vi "LEBITplc.DelayedDC.vi"(1 "i attribute":T1, 2 "Nickname":string="NDC6", 4 "Delayed DC":string[][](array[string]), 5 "Value":dbl, 8 "Enum":enum16{"RFAMP3", "Alpha", "DC"}(ring)) -> (14 "NicknamePDC":string, 15 "NicknameNDC":string, 16 "ValuePDC":dbl, 17 "IndexPDC":i32, 18 "ValueNDC":dbl, 19 "IndexNDC":i32)   [LabVIEW 2014, in "LEBITplc.lvlib"]
uses:
  LEBITplc.lvlib
  LEBITplc.i attribute.ctl
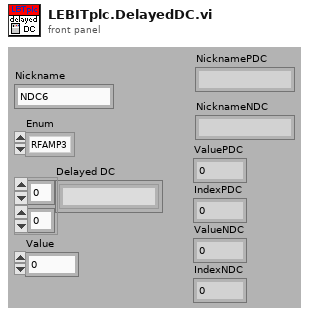
[diagram p1: front panel]
types:
  T1 = typedef "LEBITplc.lvlib/LEBITplc.i attribute.ctl" = cluster{"LLFLocation":string, "SetFileLocation":string, "nickNames":string[], "setValuePLCServiceID":i32[], "GUIServiceID":i32[], "monValuePLC":string[], "SetValueServiceID":i32[], "MonValueServiceID":i32[], "SetValue":dbl[][], "SetValueMin":dbl[], "SetValueMax":dbl[], "SetValueInfoServiceID":i32[], "GUINames":string[], "ListOfBases":string[], "Scale":dbl[], "Offset":dbl[], "setValuePLC":string[], "BaseName":string[], "ScaleServiceID":i32[], "OffsetServiceID":i32[], "AllPLCValues":string[], "CondSpecialArray":string[][], "CondSpecialIndex":i32[], "CondSpecialMonValue":dbl[], "RecentlyChanged":i32[], "SetFileLocationID":i32, "Dependent-Monitors":string[][], "LastLoadedFiles":string[], "IonGuideCalibLocation":string, "Monitor Dependent":string[], "Special":string[], "PLC?":bool[], "Start Date":string, "ListOfBasesServiceID":i32, "SETRA VISA resource":refnum<visa-resource-name>}
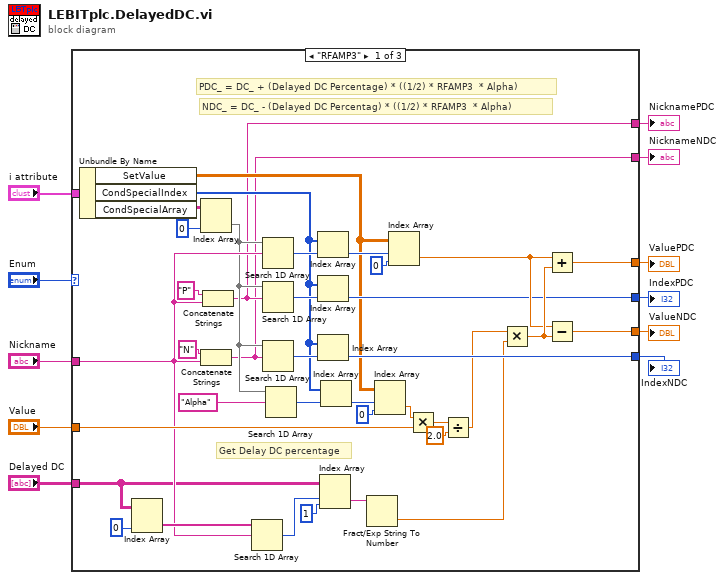
[diagram p0: block diagram]
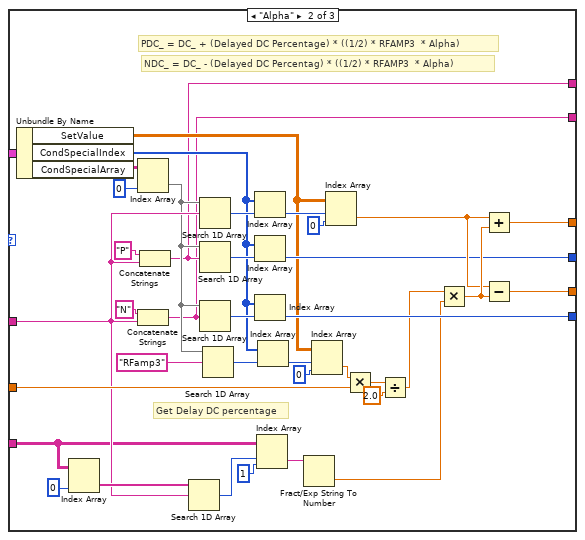
[diagram p2: hidden frame]
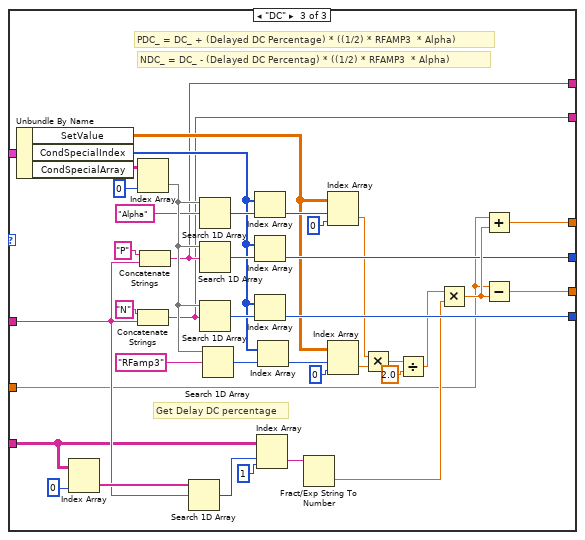
[diagram p3: hidden frame]
diagram:
  n1 = case shown="\"RFAMP3\"" "Enum" {
    tunnel: "Value" -> [w36 w74 w90]
    tunnel: [w40 w78 w118] -> w6
    tunnel: [w39 w77 w117] -> w7
    tunnel: [w38 w76 w116] -> w8
    tunnel: [w37 w75 w115] -> w9
    tunnel: "Nickname" -> [w28 w66 w107]
    tunnel: "i attribute" -> [w32 w70 w111]
    tunnel: "Delayed DC" -> [w27 w65 w106]
    tunnel: [w13 w51 w89] -> w2
    tunnel: [w12 w50 w88] -> w1
    frame "RFAMP3" {
      # "Get Delay DC percentage"
      # "NDC_ = DC_ - (Delayed DC Percentag) * ((1/2) * RFAMP3  * Alpha)"
      # "PDC_ = DC_ + (Delayed DC Percentage) * ((1/2) * RFAMP3  * Alpha)"
      n2 = Unbundle By Name(w32) -> ("SetValue"=w19:dbl[][], "CondSpecialIndex"=w23:i32[], "CondSpecialArray"=w31:string[][])
      n3 = Index Array(array=w27, index (col)=0 ("disabled index (col)")) -> (element=w29:string[])  [unwired: 1 in]
      n4 = Index Array(array=w31, index (col)=0 ("index (row)")) -> (element=w22:string[])  [unwired: 1 in]
      n5 = Concatenate Strings("N" ("string"), w28) -> (w12:string)
      n6 = Concatenate Strings("P" ("string"), w28) -> (w13:string)
      n7 = Search 1D Array(1D array=w29, element=w28) -> (index of element=w25:i32)  [unwired: 1 in]
      n8 = Search 1D Array(1D array=w22, element=w28) -> (index of element=w46:i32)  [unwired: 1 in]
      n9 = Search 1D Array(1D array=w22, element=w13) -> (index of element=w47:i32)  [unwired: 1 in]
      n10 = Search 1D Array(1D array=w22, element=w12) -> (index of element=w48:i32)  [unwired: 1 in]
      n11 = Search 1D Array(1D array=w22, element="Alpha") -> (index of element=w24:i32)  [unwired: 1 in]
      n12 = Index Array(array=w23, index=w46) -> (element=w44:i32)
      n13 = Index Array(array=w23, index=w47) -> (element=w39:i32)
      n14 = Index Array(array=w23, index=w48) -> (element=w37:i32)
      n15 = Index Array(array=w27, index (row)=w25, index (col)=1 ("disabled index (col)")) -> (element=w15:string)
      n16 = Index Array(array=w23, index=w24) -> (element=w18:i32)
      n17 = Fract/Exp String To Number(string=w15) -> (number=w14:dbl)  [unwired: 3 in, 1 out]
      n18 = Index Array(array=w19, index (row)=w18, index (col)=0 ("disabled index (col)")) -> (element=w17:dbl)
      n19 = Index Array(array=w19, index (row)=w44, index (col)=0 ("disabled index (col)")) -> (element=w43:dbl)
      n20 = Multiply(x=w17, y=w36) -> (x*y=w42:dbl)
      n21 = Divide(x=w42, y=2.0) -> (x/y=w16:dbl)
      n22 = Multiply(x=w16, y=w14) -> (x*y=w49:dbl)
      n23 = Add(x=w43, y=w49) -> (x+y=w40:dbl)
      n24 = Subtract(x=w43, y=w49) -> (x-y=w38:dbl)
    }
    frame "Alpha" {
      # "Get Delay DC percentage"
      # "NDC_ = DC_ - (Delayed DC Percentag) * ((1/2) * RFAMP3  * Alpha)"
      # "PDC_ = DC_ + (Delayed DC Percentage) * ((1/2) * RFAMP3  * Alpha)"
      n25 = Unbundle By Name(w70) -> ("SetValue"=w57:dbl[][], "CondSpecialIndex"=w61:i32[], "CondSpecialArray"=w69:string[][])
      n26 = Index Array(array=w65, index (col)=0 ("disabled index (col)")) -> (element=w67:string[])  [unwired: 1 in]
      n27 = Index Array(array=w69, index (col)=0 ("index (row)")) -> (element=w60:string[])  [unwired: 1 in]
      n28 = Concatenate Strings("N" ("string"), w66) -> (w50:string)
      n29 = Concatenate Strings("P" ("string"), w66) -> (w51:string)
      n30 = Search 1D Array(1D array=w67, element=w66) -> (index of element=w63:i32)  [unwired: 1 in]
      n31 = Search 1D Array(1D array=w60, element=w66) -> (index of element=w84:i32)  [unwired: 1 in]
      n32 = Search 1D Array(1D array=w60, element=w51) -> (index of element=w85:i32)  [unwired: 1 in]
      n33 = Search 1D Array(1D array=w60, element=w50) -> (index of element=w86:i32)  [unwired: 1 in]
      n34 = Search 1D Array(1D array=w60, element="RFamp3") -> (index of element=w62:i32)  [unwired: 1 in]
      n35 = Index Array(array=w61, index=w84) -> (element=w82:i32)
      n36 = Index Array(array=w61, index=w85) -> (element=w77:i32)
      n37 = Index Array(array=w61, index=w86) -> (element=w75:i32)
      n38 = Index Array(array=w65, index (row)=w63, index (col)=1 ("disabled index (col)")) -> (element=w53:string)
      n39 = Index Array(array=w61, index=w62) -> (element=w56:i32)
      n40 = Fract/Exp String To Number(string=w53) -> (number=w52:dbl)  [unwired: 3 in, 1 out]
      n41 = Index Array(array=w57, index (row)=w56, index (col)=0 ("disabled index (col)")) -> (element=w55:dbl)
      n42 = Index Array(array=w57, index (row)=w82, index (col)=0 ("disabled index (col)")) -> (element=w81:dbl)
      n43 = Multiply(x=w55, y=w74) -> (x*y=w80:dbl)
      n44 = Divide(x=w80, y=2.0) -> (x/y=w54:dbl)
      n45 = Multiply(x=w54, y=w52) -> (x*y=w87:dbl)
      n46 = Add(x=w81, y=w87) -> (x+y=w78:dbl)
      n47 = Subtract(x=w81, y=w87) -> (x-y=w76:dbl)
    }
    frame "DC" {
      # "Get Delay DC percentage"
      # "NDC_ = DC_ - (Delayed DC Percentag) * ((1/2) * RFAMP3  * Alpha)"
      # "PDC_ = DC_ + (Delayed DC Percentage) * ((1/2) * RFAMP3  * Alpha)"
      n48 = Unbundle By Name(w111) -> ("SetValue"=w98:dbl[][], "CondSpecialIndex"=w102:i32[], "CondSpecialArray"=w110:string[][])
      n49 = Index Array(array=w106, index (col)=0 ("disabled index (col)")) -> (element=w108:string[])  [unwired: 1 in]
      n50 = Index Array(array=w110, index (col)=0 ("index (row)")) -> (element=w101:string[])  [unwired: 1 in]
      n51 = Concatenate Strings("N" ("string"), w107) -> (w88:string)
      n52 = Concatenate Strings("P" ("string"), w107) -> (w89:string)
      n53 = Search 1D Array(1D array=w108, element=w107) -> (index of element=w104:i32)  [unwired: 1 in]
      n54 = Search 1D Array(1D array=w101, element="Alpha") -> (index of element=w123:i32)  [unwired: 1 in]
      n55 = Search 1D Array(1D array=w101, element=w89) -> (index of element=w124:i32)  [unwired: 1 in]
      n56 = Search 1D Array(1D array=w101, element=w88) -> (index of element=w125:i32)  [unwired: 1 in]
      n57 = Search 1D Array(1D array=w101, element="RFamp3") -> (index of element=w103:i32)  [unwired: 1 in]
      n58 = Index Array(array=w102, index=w123) -> (element=w121:i32)
      n59 = Index Array(array=w102, index=w124) -> (element=w117:i32)
      n60 = Index Array(array=w102, index=w125) -> (element=w115:i32)
      n61 = Index Array(array=w106, index (row)=w104, index (col)=1 ("disabled index (col)")) -> (element=w95:string)
      n62 = Index Array(array=w102, index=w103) -> (element=w97:i32)
      n63 = Fract/Exp String To Number(string=w95) -> (number=w94:dbl)  [unwired: 3 in, 1 out]
      n64 = Index Array(array=w98, index (row)=w121, index (col)=0 ("disabled index (col)")) -> (element=w92:dbl)
      n65 = Index Array(array=w98, index (row)=w97, index (col)=0 ("disabled index (col)")) -> (element=w91:dbl)
      n66 = Multiply(x=w92, y=w91) -> (x*y=w120:dbl)
      n67 = Divide(x=w120, y=2.0) -> (x/y=w96:dbl)
      n68 = Multiply(x=w96, y=w94) -> (x*y=w126:dbl)
      n69 = Add(x=w90, y=w126) -> (x+y=w118:dbl)
      n70 = Subtract(x=w90, y=w126) -> (x-y=w116:dbl)
    }
  }
  "IndexNDC" <- w9
  "IndexPDC" <- w7
  "ValueNDC" <- w8
  "ValuePDC" <- w6
  "NicknamePDC" <- w2
  "NicknameNDC" <- w1
